vi "cblas zaxpy.vi"(5 "n":i32=-1, 6 "incy":i32=1, 7 "incx":i32=1, 9 "alpha":cdb=1.0+0.0i, 10 "y":cdb[](array[numeric]), 11 "x":cdb[](array[numeric])) -> (0 "error":i32, 3 "zaxpy":cdb[](array[numeric]))   [LabVIEW 2017, in "NI_AALBLAS.lvlib"]
uses:
  <vilib>/Analysis/NI_AALBLAS.lvlib
  <resource>/lvblas.dll
panel:
  # "void cblas_zaxpy(n, *alpha, *x, incx, *y, incy)"
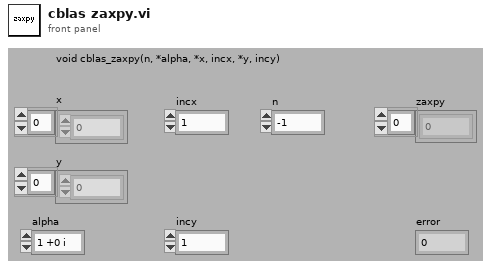
[diagram p1: front panel]
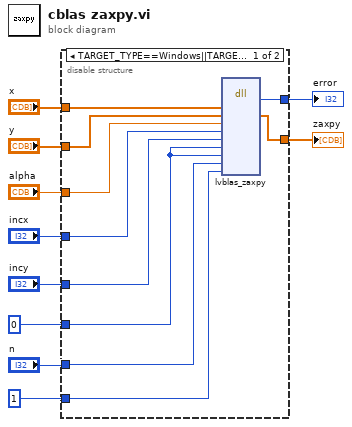
[diagram p0: block diagram]
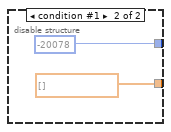
[diagram p2: hidden frame]
diagram:
  n1 = disable-structure shown="TARGET_TYPE==Windows||TARGET_TYPE==Unix||TARGET_TYPE==RT||TARGET_TYPE==Mac" {
    disable-tunnel: "x" -> [w20 _]
    disable-tunnel: "y" -> [w19 _]
    disable-tunnel: [w18 -20078] -> w10
    disable-tunnel: "alpha" -> [w17 _]
    disable-tunnel: "n" -> [w16 _]
    disable-tunnel: [w15 cdb[] []] -> w5
    disable-tunnel: 0 -> [w14 _]
    disable-tunnel: "incx" -> [w13 _]
    disable-tunnel: "incy" -> [w12 _]
    disable-tunnel: 1 -> [w11 _]
    frame condition #0 (active) {
      n2 = dll-call lib="e:/builds/penguin/labview/branches/2017/dev/dist/resource/lvblas.*" fn="lvblas_zaxpy" ("CBLAS.dll:DotProdH")("X"=w20, "Y"=w19, "alpha"=w17, "IncX"=w13, "IncY"=w12, "startX"=w14, "startY"=w14, "N"=w16, "check"=w11) -> ("error"=w18:i32, "Y"=w15:cdb[])  [unwired: 11 in, 2 out]
    }
    frame condition #1 {
    }
  }
  "zaxpy" <- w5
  "error" <- w10
